vi "测量计算.vi"(11 "Dynamic Data输入":dynamicdata(waveform) caption="Dynamic Data") -> (3 "Dynamic Data输出":dynamicdata(waveform) caption="Dynamic Data")   [LabVIEW 2016]
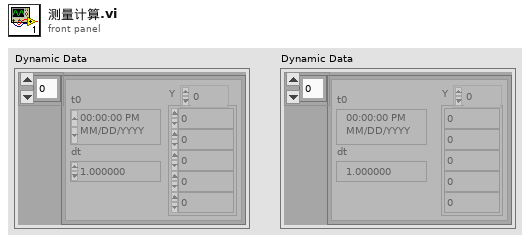
[diagram p1: front panel]
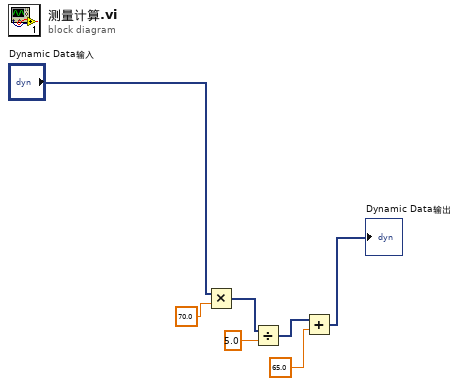
[diagram p0: block diagram]
diagram:
  n1 = Multiply(x="Dynamic Data输入", y=70.0) -> (x*y=w3:dynamicdata)
  n2 = Divide(x=w3, y=5.0) -> (x/y=w5:dynamicdata)
  n3 = Add(x=w5, y=65.0) -> (x+y=→"Dynamic Data输出":dynamicdata)
